vi "Get_Status.vi"(7 "I2C Channel":u8, 8 "error in":errorcluster, 11 "LINX Resource In":T2) -> (0 "error out":errorcluster, 2 "Device Status":T1, 3 "LINX Resource Out":T2)   [LabVIEW 2014, in "LMH-LINX.lvlib" / "LIS331HH.lvlib"]
doc: "This VI reads the status register of the device to provide information about Accelerometer data availability\n\n**Author: Stas Legedza"
uses:
  <vilib>/MakerHub/LINX/Public/Sensors/Accelerometer/LIS331HH/LIS331HH.lvlib
  <vilib>/MakerHub/LINX/Private/Type Defs/LINX Ref.ctl
  <vilib>/MakerHub/LINX/Private/Type Defs/Platform.ctl
  <vilib>/MakerHub/LINX/Private/Type Defs/Interface.ctl
  <vilib>/MakerHub/LINX/Private/Device/Type Defs/LINX Device Config.ctl
  <vilib>/MakerHub/LINX/Private/Device/Type Defs/TCP Config.ctl
  <vilib>/MakerHub/LINX/Private/Device/Type Defs/Channels.ctl
  <vilib>/MakerHub/LINX/Public/Sensors/Accelerometer/LIS331HH/Controls/Status_Register.ctl
  <vilib>/MakerHub/LINX/LMH-LINX.lvlib
  <vilib>/MakerHub/LINX/Private/Device/Device.lvlib
panel:
  # "INPUTS"
  # "OUTPUTS"
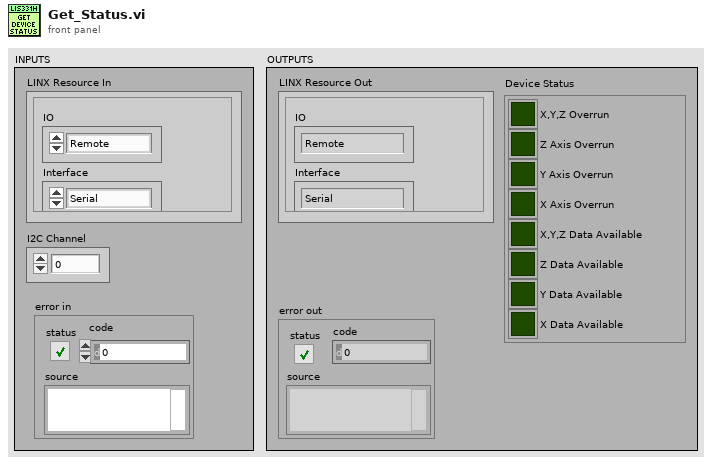
[diagram p1: front panel]
types:
  T1 = typedef "LMH-LINX.lvlib/LIS331HH.lvlib/Status_Register.ctl" = cluster{"X,Y,Z Overrun":bool, "Z Axis Overrun":bool, "Y Axis Overrun":bool, "X Axis Overrun":bool, "X,Y,Z Data Available":bool, "Z Data Available":bool, "Y Data Available":bool, "X Data Available":bool}
  T2 = typedef "LMH-LINX.lvlib/LINX Ref.ctl" = cluster{"IO":T3, "Interface":T4, "LINX Device Config":T5}
  T3 = typedef "LMH-LINX.lvlib/Platform.ctl" = enum16{"Remote", "Local"}
  T4 = typedef "LMH-LINX.lvlib/Interface.ctl" = enum16{"Serial", "TCP"}
  T5 = typedef "LMH-LINX.lvlib/Device.lvlib/LINX Device Config.ctl" = cluster{"Interface":T4, "COM Port":refnum<visa-resource-name>, "TCP Configuration":T6, "Device Family":u8, "Device ID":u8, "Device Name":string, "TCP Ref":refnum<k5>, "Channels":T7}
  T6 = typedef "LMH-LINX.lvlib/Device.lvlib/TCP Config.ctl" = cluster{"IP Address":string, "Port":u16}
  T7 = typedef "LMH-LINX.lvlib/Channels.ctl" = cluster{"DI":u8[], "DO":u8[], "AI":u8[], "AO":u8[], "PWM":u8[], "QE":u8[], "UART":u8[], "I2C 2":u8[], "SPI":u8[], "CAN":u8[], "Servo":u8[], "AI Ref (V)":dbl, "AI Resolution (Bits)":u8, "AO Ref (V)":dbl, "AO Resolution (Bits)":u8}
  T8 = cluster{"Boolean array[0]":bool, "Boolean array[1]":bool, "Boolean array[2]":bool, "Boolean array[3]":bool, "Boolean array[4]":bool, "Boolean array[5]":bool, "Boolean array[6]":bool, "Boolean array[7]":bool}
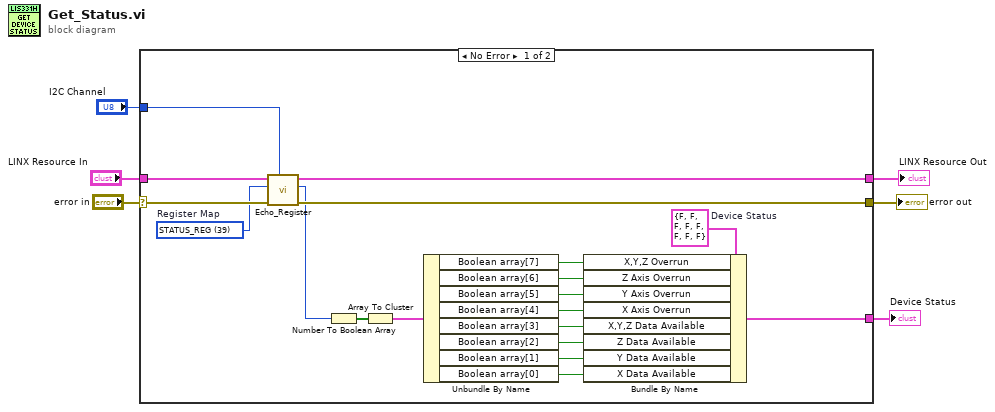
[diagram p0: block diagram]
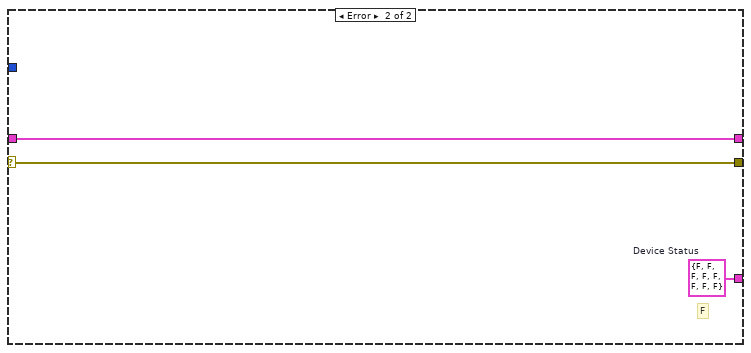
[diagram p2: hidden frame]
diagram:
  n1 = case shown="No Error" "error in" {
    selector: "error in" -> [w24 w28]
    tunnel: [w20 w28] -> w5
    tunnel: "LINX Resource In" -> [w25 w27]
    tunnel: "I2C Channel" -> [w23 _]
    tunnel: [w21 w27] -> w2
    tunnel: [w18 w26] -> w1
    frame No Error {
      w19 = T1 {"X,Y,Z Overrun"=FALSE, "Z Axis Overrun"=FALSE, "Y Axis Overrun"=FALSE, "X Axis Overrun"=FALSE, "X,Y,Z Data Available"=FALSE, "Z Data Available"=FALSE, "Y Data Available"=FALSE, "X Data Available"=FALSE}  # Device Status
      w22 = u8 39 items=["CTRL_REG1"=32, "CTRL_REG2"=33, "CTRL_REG3"=34, "CTRL_REG4"=35, "CTRL_REG5"=36, "HP_FILTER_RESET"=37, "REFERENCE"=38, "STATUS_REG"=39, "OUT_X_L"=40, "OUT_X_H"=41, "OUT_Y_L"=42, "OUT_Y_H"=43, "OUT_Z_L"=44, "OUT_Z_H"=45, "INT1_CFG"=48, "INT1_SOURCE"=49, "INT1_THS"=50, "INT1_DURATION"=51, "INT2_CFG"=52, "INT2_SOURCE"=53, "INT2_THS"=54, "INT2_DURATION"=55]  # Register Map
      n2 = call <vilib>:"Echo_Register.vi"("I2C Channel"=w23, "error in (no error)"=w24, "Register to Echo"=w22, "LINX Resource In"=w25) -> ("error out"=w20:errorcluster, "Register Word"=w16:u8, "LINX Resource Out"=w21:T2)  [unwired: 5 in]
      n3 = Number To Boolean Array(number=w16) -> (Boolean array=w17:bool[])
      n4 = Array To Cluster(array=w17) -> (cluster=w15:T8)
      n5 = Unbundle By Name(w15) -> ("Boolean array[7]"=w14:bool, "Boolean array[6]"=w13:bool, "Boolean array[5]"=w12:bool, "Boolean array[4]"=w11:bool, "Boolean array[3]"=w10:bool, "Boolean array[2]"=w9:bool, "Boolean array[1]"=w8:bool, "Boolean array[0]"=w7:bool)
      n6 = Bundle By Name(cluster=w19, "X,Y,Z Overrun"=w14, "Z Axis Overrun"=w13, "Y Axis Overrun"=w12, "X Axis Overrun"=w11, "X,Y,Z Data Available"=w10, "Z Data Available"=w9, "Y Data Available"=w8, "X Data Available"=w7) -> (w18:T1)
    }
    frame Error {
      w26 = T1 {"X,Y,Z Overrun"=FALSE, "Z Axis Overrun"=FALSE, "Y Axis Overrun"=FALSE, "X Axis Overrun"=FALSE, "X,Y,Z Data Available"=FALSE, "Z Data Available"=FALSE, "Y Data Available"=FALSE, "X Data Available"=FALSE}  # Device Status
      # "F"
    }
  }
  "error out" <- w5
  "LINX Resource Out" <- w2
  "Device Status" <- w1
